vi "FRCts20_Backend_API_S3.vi"(8 "error in (no error)":errorcluster, 10 "Temporary URL":string, 11 "Team Index":u32) -> (0 "error out":errorcluster, 2 "Status":string, 3 "S3":T1)   [LabVIEW 2014]
doc: "This VI could be in charge of controlling the backend, but at present it is not."
uses:
  FRCts20_Backend_FGVOperation.ctl
  FRCts20_Backend_Engine.lvlib
  FRCts20_Backend_API_S3.ctl
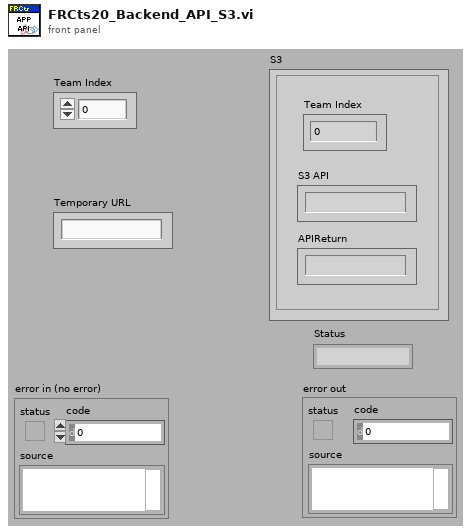
[diagram p1: front panel]
types:
  T1 = typedef "FRCts20_Backend_API.lvlib/FRCts20_Backend_API_S3.ctl" = cluster{"S3 API":string, "APIReturn":string, "Team Index":u32}
  T2 = typedef "FRCts20_Backend_Engine.lvlib/FRCts20_Backend_FGVOperation.ctl" = enum16{"Initialize", "EnqueueMessage", "EnqueueDataReturn", "FlushMessage", "FlushDataReturn"}
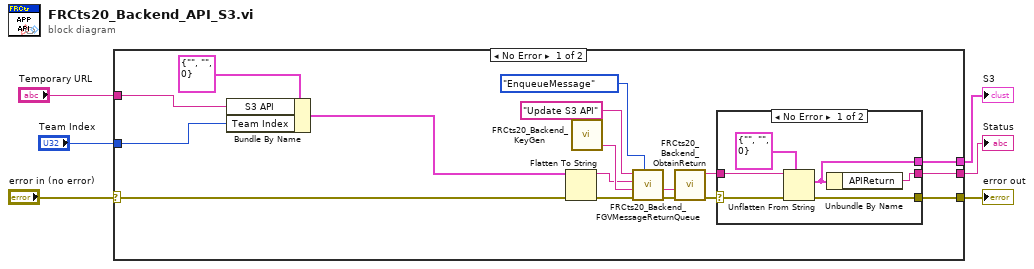
[diagram p0: block diagram]
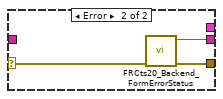
[diagram p2: hidden frame]
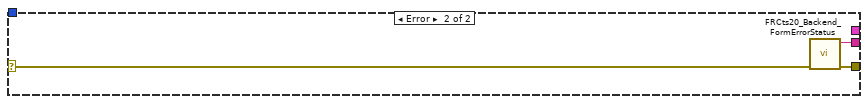
[diagram p3: hidden frame]
diagram:
  n1 = case shown="No Error" "error in (no error)" {
    selector: "error in (no error)" -> [w7 w35]
    tunnel: [w16 w34] -> w5
    tunnel: [w14 w33] -> w4
    tunnel: [w15 _] -> w3
    tunnel: "Temporary URL" -> [w9 _]
    tunnel: "Team Index" -> [w8 _]
    frame No Error {
      n2 = Bundle By Name(cluster=T1 {"S3 API"="", "APIReturn"="", "Team Index"=0} ("S3"), "S3 API"=w9, "Team Index"=w8) -> (w10:T1)
      n3 = Flatten To String(anything=w10, error in (no error)=w7) -> (data string=w18:string, error out=w19:errorcluster)  [unwired: 2 in, 1 out]
      n4 = call "FRCts20_Backend_KeyGen.vi"() -> ("Keygen"=w23:string)  [unwired: 27 in]
      n5 = call "FRCts20_Backend_FGVMessageReturnQueue.vi"("Operation"=FRCts20_Backend_FGVOperation."EnqueueMessage", "error in (no error)"=w19, "Key"=w23, "Message Value"=w18, "Message Name"="Update S3 API") -> ("error out"=w21:errorcluster, "Key (Duplicate)"=w20:string)  [unwired: 5 in]
      n6 = call "FRCts20_Backend_ObtainReturn.vi"("error in (no error)"=w21, "Key"=w20) -> ("error out"=w17:errorcluster, "Message Value"=w13:string)  [unwired: 8 in]
      n7 = case shown="No Error" w17 {
        selector: w17 -> [w28 w31]
        tunnel: [w29 w32] -> w16
        tunnel: [w27 _] -> w15
        tunnel: [w26 w30] -> w14
        tunnel: w13 -> [w25 _]
        frame No Error {
          n8 = Unflatten From String(type=T1 {"S3 API"="", "APIReturn"="", "Team Index"=0} ("S3"), binary string=w25, error in (no error)=w28) -> (value=w27:T1, error out=w29:errorcluster)  [unwired: 2 in, 1 out]
          n9 = Unbundle By Name(w27) -> ("APIReturn"=w26:string)
        }
        frame Error {
          n10 = call "FRCts20_Backend_FormErrorStatus.vi"("error in (no error)"=w31) -> ("error out"=w32:errorcluster, "String"=w30:string)  [unwired: 9 in]
        }
      }
    }
    frame Error {
      n11 = call "FRCts20_Backend_FormErrorStatus.vi"("error in (no error)"=w35) -> ("error out"=w34:errorcluster, "String"=w33:string)  [unwired: 9 in]
    }
  }
  "error out" <- w5
  "Status" <- w4
  "S3" <- w3
